vi "Read Array of Port Sessions.vi"(8 "error in":errorcluster, 11 "port node in":refnum<k20>) -> (0 "error out":errorcluster, 2 "session type":string[](array[string]), 3 "port node out":refnum<k20>[](array[refnum]))   [LabVIEW 2020, in "AIM ARINC 664 Import.lvlib"]
uses:
  AIM ARINC 664 Import.lvlib
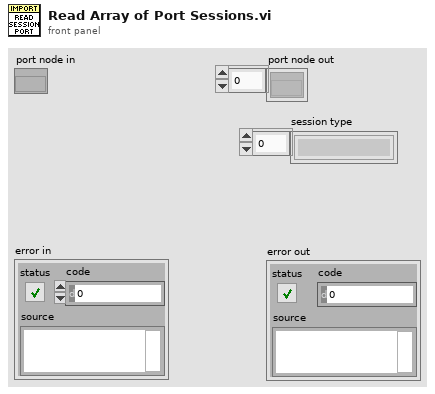
[diagram p1: front panel]
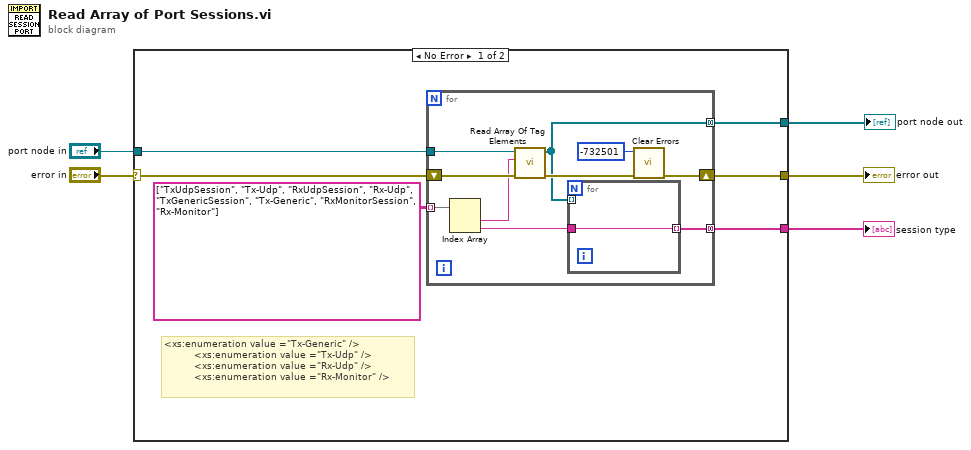
[diagram p0: block diagram]
diagram:
  n1 = case shown="No Error" "error in" {
    selector: "error in" -> [w11 w23]
    tunnel: [w7 w23] -> w5
    tunnel: "port node in" -> [w10 _]
    tunnel: [w9 _] -> w3
    tunnel: [w6 _] -> w1
    frame No Error {
      # "<xs:enumeration value =\"Tx-Generic\" />\n          <xs:enumeration value =\"Tx-Udp\" />\n          <xs:enumeration value =\"Rx-Udp\" />\n          <xs:enumeration value =\"Rx-Monitor\" />"
      n2 = for {
        tunnel: w10 -> [w20]
        tunnel: [w18] -> w9 mode=concatenating
        tunnel: string[][] [["TxUdpSession", "Tx-Udp"], ["RxUdpSession", "Rx-Udp"], ["TxGenericSession", "Tx-Generic"], ["RxMonitorSession", "Rx-Monitor"]] -> [w15] mode=indexing
        shift-right: [w17] -> w7
        shift-left: w11 -> [w21]
        tunnel: [w13] -> w6 mode=concatenating
        n3 = Index Array(array=w15) -> (element #1=w14:string, element #2=w12:string)  [unwired: 2 in]
        n4 = call "Read Array Of Tag Elements.vi"("error in"=w21, "tag name"=w14, "node in"=w20) -> ("error out"=w19:errorcluster, "array of elements"=w18:refnum<k20>[])  [unwired: 7 in]
        n5 = for {
          tunnel: w18 -> [_] mode=indexing
          tunnel: [w22] -> w13 mode=indexing
          tunnel: w12 -> [w22]
        }
        n6 = call <vilib>:"Clear Errors.vi"("error in (no error)"=w19, "specific error code to clear (0: all)"=-732501) -> ("error out"=w17:errorcluster)  [unwired: 4 in, 1 out]
      }
    }
    frame Error {
    }
  }
  "error out" <- w5
  "port node out" <- w3
  "session type" <- w1
